vi "Lauda Test Program.vi"() -> ()   [LabVIEW 2018, in "Lauda TCU.lvlib"]
uses:
  Lauda TCU.lvlib
  Lauda Settings.ctl
  <vilib>/Platform/TimedLoop/XDataNode/timing_clust.ctl
  <vilib>/Platform/TimedLoop/XDataNode/nitl_modes.ctl
  <vilib>/Platform/TimedLoop/XDataNode/wakeup.ctl
  <vilib>/Platform/TimedLoop/XDataNode/XDataNode.xnode
  support/Support Library.lvlib
  <vilib>/Platform/TimedLoop/XDataNode/XDNodeRunTimeDep.lvlib
panel:
  out "Running":bool
  out "Connection Error":bool
  in  "stop":bool
  in  "Temp":dbl
  in  "Run":bool
  out "error out":errorcluster
  in  "error in (no error)":errorcluster
  out "Huber Settings":T1
  in  "Huber Settings":T1
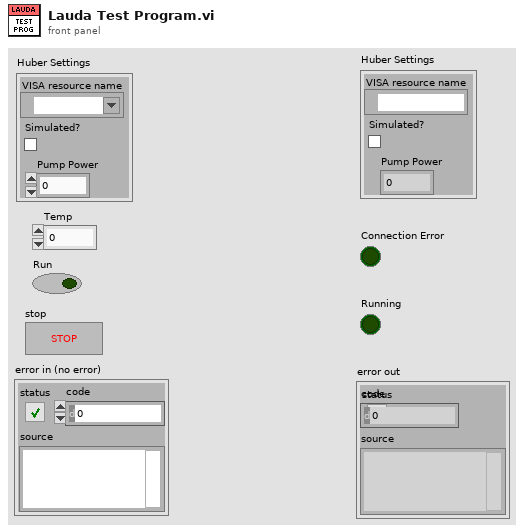
[diagram p1: front panel]
types:
  T1 = typedef "Lauda TCU.lvlib/Lauda Settings.ctl" = cluster{"VISA resource name":refnum<visa-resource-name>, "Simulated?":bool, "Pump Power":i32}
  T2 = typedef "XDNodeRunTimeDep.lvlib/timing_clust.ctl" = cluster{"Expected End [f-1]":u64, "Actual End [f-1]":u64, "Finished Late? [f-1]":bool, "Expected End [i-1]":u64, "Actual End [i-1]":u64, "Finished Late? [i-1]":bool, "Expected Start [i]":u64, "Actual Start [i]":u64, "Expected Start [f]":u64, "Actual Start [f]":u64, "Source Name":string, "Structure Name":string, "Period":i64, "Deadline":i64, "Offset":i64, "Start":i64, "Priority":i32, "Timeout":i32, "Mode":T3, "Wakeup Reason":T4, "Error":errorcluster, "Source Type":string, "Secondary Source Type":string, "Global End Time":u64, "Global Start Time":u64, "Frame Duration":u64, "Iteration Duration":u64, "Assigned CPU":i32, "I/O Scan Engine Mode":u32}
  T3 = typedef "XDNodeRunTimeDep.lvlib/nitl_modes.ctl" = enum32{"No Change", "Process missed periods, maintain original phase", "Discard missed periods, maintain original phase", "Process missed periods, ignore original phase", "Discard missed periods, ignore original phase"}
  T4 = typedef "XDNodeRunTimeDep.lvlib/wakeup.ctl" = enum32{"Normal", "Aborted", "Asynchronous wakeup", "Timing source error", "Timed loop error", "Timeout"}
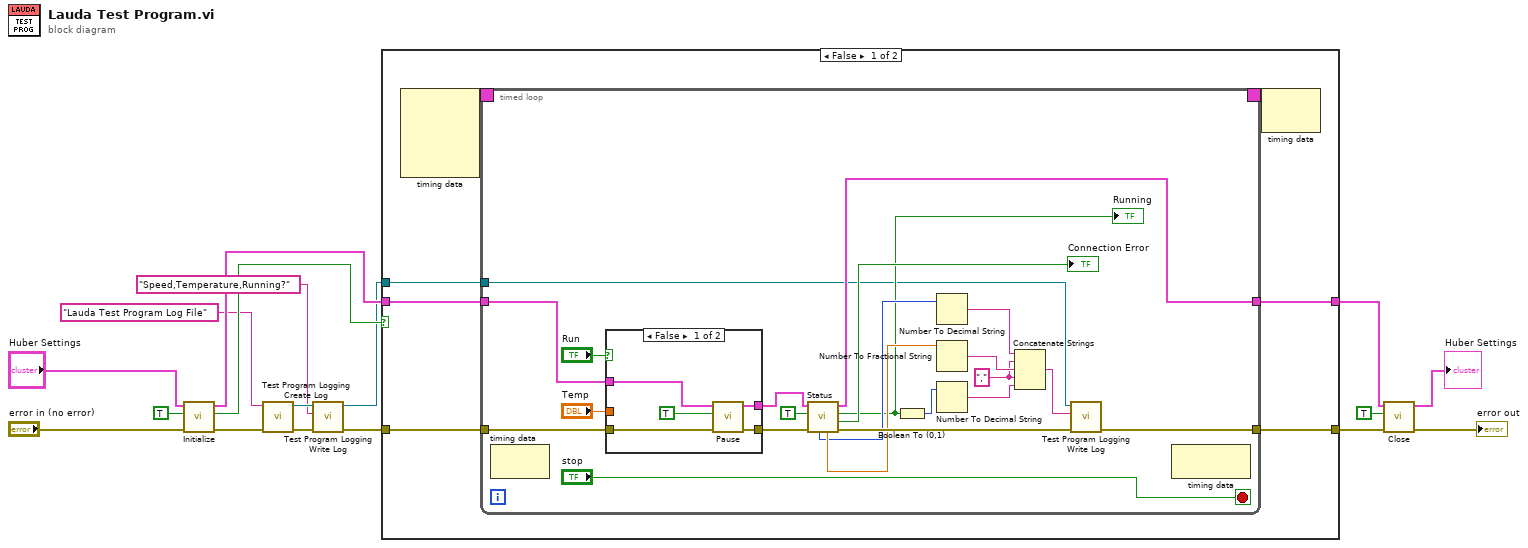
[diagram p0: block diagram]
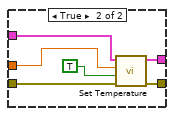
[diagram p2: hidden frame]
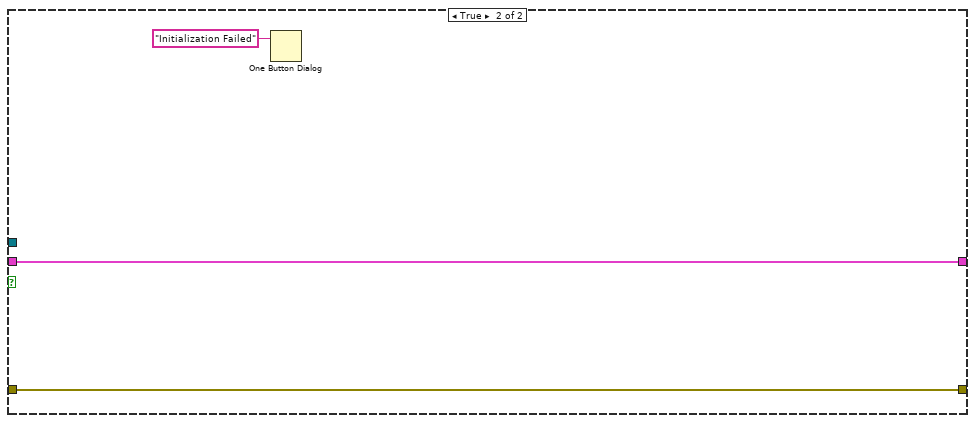
[diagram p3: hidden frame]
diagram:
  n1 = call "Initialize.vi"("error in (no error)"="error in (no error)", "Internal?"=TRUE, "Lauda Settings In"="Huber Settings") -> ("error out"=w6:errorcluster, "Connection Error"=w10:bool, "Lauda Settings Out"=w11:T1)  [unwired: 6 in]
  n2 = call "Test Program Logging Create Log.vi"("error in"=w6, "string"="Lauda Test Program Log File") -> ("error out"=w5:errorcluster, "refnum out"=w3:refnum<file>)  [unwired: 8 in]
  n3 = call "Test Program Logging Write Log.vi"("error in"=w5, "text"="Speed,Temperature,Running?", "Test Program Log File"=w3) -> ("error out"=w4:errorcluster, "refnum out"=w1:refnum<file>)  [unwired: 7 in]
  n4 = case shown="False" w10 {
    tunnel: [w24 w63] -> w15
    tunnel: [w23 w62] -> w13
    tunnel: w11 -> [w22 w63]
    tunnel: w4 -> [w21 w62]
    tunnel: w1 -> [w18 _]
    frame False {
      n5 = node-c288() -> (w20:T2)  [unwired: 4 in]
      n6 = timed-loop {
        tunnel: [w46] -> w24
        tunnel: [w36] -> w23
        tunnel: w22 -> [w44]
        tunnel: w21 -> [w43]
        timing: w20 -> [_]
        timing-out: [_] -> w19
        tunnel: w18 -> [w26]
        stop <- "stop" stop-if-true
        w27 = "," ("string")
        n7 = node-c288() -> ()  [unwired: 1 in, 1 out]
        n8 = case shown="False" "Run" {
          tunnel: w44 -> [w53 w59]
          tunnel: w43 -> [w52 w58]
          tunnel: [w51 w57] -> w42
          tunnel: [w50 w56] -> w41
          tunnel: "Temp" -> [_ w55]
          frame False {
            n9 = call "Pause.vi"("error in (no error)"=w52, "Internal?"=TRUE, "Huber Settings In"=w53) -> ("error out"=w51:errorcluster, "Huber Settings Out"=w50:T1)  [unwired: 7 in]
          }
          frame True {
            n10 = call "Set Temperature.vi"("error in (no error)"=w58, "Internal?"=TRUE, "Setpoint"=w55, "Lauda Settings In"=w59) -> ("error out"=w57:errorcluster, "Lauda Settings Out"=w56:T1)  [unwired: 5 in, 1 out]
          }
        }
        n11 = call "Status.vi"("error in (no error)"=w42, "Internal?"=TRUE, "Lauda Settings"=w41) -> ("error out"=w37:errorcluster, "Connection Error"=→"Connection Error":bool, "Running"=w31:bool, "Lauda Settings"=w46:T1, "Temp"=w34:dbl, "Pump Speed"=w33:i32)  [unwired: 2 in, 1 out]
        "Running" <- w31
        n12 = Boolean To (0,1)(Boolean=w31) -> (0, 1=w32:i16)
        n13 = Number To Decimal String(number=w33) -> (decimal integer string=w30:string)  [unwired: 1 in]
        n14 = Number To Fractional String(number=w34) -> (F-format string=w28:string)  [unwired: 3 in]
        n15 = Number To Decimal String(number=w32) -> (decimal integer string=w29:string)  [unwired: 1 in]
        n16 = Concatenate Strings(w30, w27, w28, w27, w29) -> (w25:string)
        n17 = call "Test Program Logging Write Log.vi"("error in"=w37, "text"=w25, "Test Program Log File"=w26) -> ("error out"=w36:errorcluster)  [unwired: 7 in, 1 out]
        n18 = node-c288() -> ()  [unwired: 1 in, 1 out]
      }
      n19 = node-c288(w19) -> ()  [unwired: 1 out]
    }
    frame True {
      n20 = One Button Dialog(message="Initialization Failed") -> ()  [unwired: 1 in, 1 out]
    }
  }
  n21 = call "Close.vi"("error in (no error)"=w13, "Internal?"=TRUE, "Lauda  Settings"=w15) -> ("error out"=→"error out":errorcluster, "Lauda Settings"=→"Huber Settings":T1)  [unwired: 7 in]
